vi "Online Spectrogram Monitoring (Simulated).vi"() -> ()   [LabVIEW 2023]
doc: "This example continuously simulates a signal and computes the real-time STFT spectrogram with the TFA Online STFT Spectrogram VI.\n\n<b>Instructions:</b>\n1) Run this VI.\n2) Observe the <b>Spectrogram</b>.\n3) Browse the Block Diagram of this example to learn how to configure the charts."
uses:
  <vilib>/addons/Time Frequency Analysis/Spectrogram.llb/TFA Online STFT Spectrogram (Real).vi
  <vilib>/addons/Time Frequency Analysis/_control.llb/TFA Configure Spectrogram Indicator (Predefined Color Table).vi
  <vilib>/addons/_Advanced Signal Processing/NI_AdvSigProcTFA.lvlib
panel:
  out "Signal":dbl[](graph)
  out "aspt-left-top":bool
  in  "Reset":bool
  in  "Stop":bool
  out "Spectrogram":dbl[][](graph)
  # "Overview: Continuously simulates a signal and computes the real-time STFT spectrogram with the TFA Online STFT Spectrogram VI.\nRequirements: LabVIEW Full Development System, Advanced Signal Processing Toolkit\nInstructions: \n1. Run this VI.\n2. Observe the Spectrogram.\n3. Browse the block diagram of this example to learn how to configure the charts.\n4. Click Stop to stop the VI."
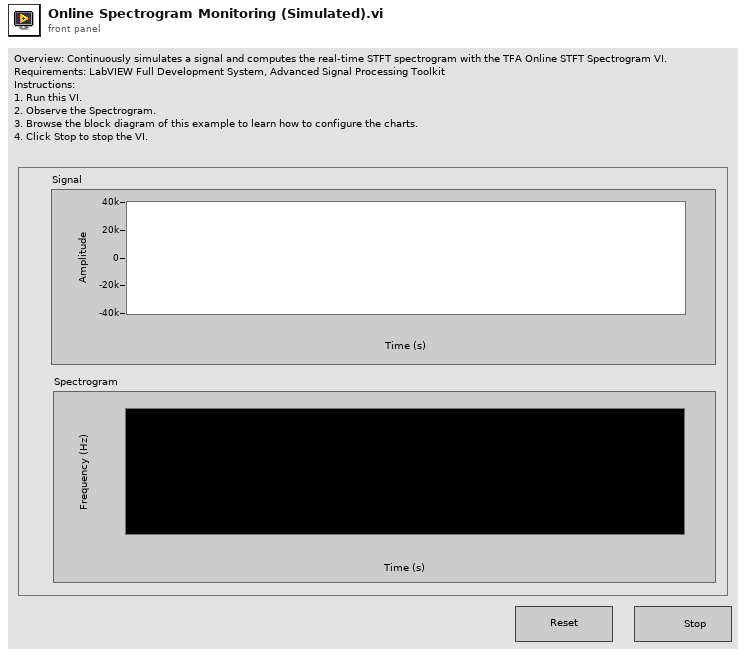
[diagram p1: front panel]
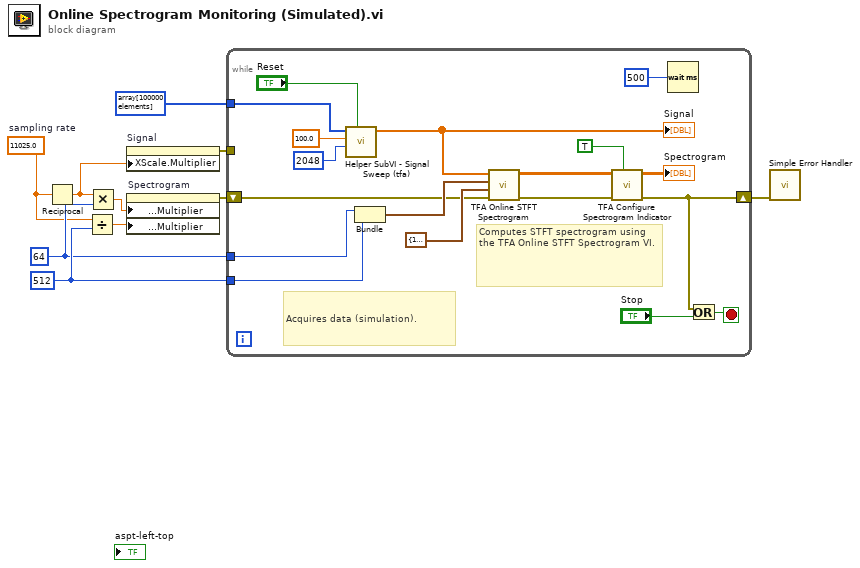
[diagram p0: block diagram]
diagram:
  w7 = 11025.0  # sampling rate
  w10 = 512 ("Frequency bins")
  w8 = 64 ("Time steps")
  n1 = Reciprocal(x=w7) -> (1/x=w4:dbl)
  n2 = Divide(x=w7, y=w10) -> (x/y=w9:dbl)
  n3 = Multiply(x=w4, y=w8) -> (x*y=w5:dbl)
  n4 = property on="Signal" class="WFChart (strict)"("XScale.Multiplier"=w4) -> (error out=w3:errorcluster)  [unwired: 2 in, 1 out]
  n5 = property on="Spectrogram" class="IntChart (strict)"("X Scale.Offset and Multiplier:Multiplier"=w5, "Y Scale.Offset and Multiplier:Multiplier"=w9) -> (error out=w6:errorcluster)  [unwired: 2 in, 1 out]
  n6 = while {
    tunnel: w8 -> [w24]
    tunnel: w10 -> [w23]
    tunnel: i16[] array[100000 elements] ("subarray") -> [w19]
    tunnel: w3 -> [_]
    shift-right: [w13] -> w2
    shift-left: w6 -> [w14]
    stop <- w11 stop-if-true
    # "Computes STFT spectrogram using the TFA Online STFT Spectrogram VI."
    # "Acquires data (simulation)."
    n7 = call "Helper SubVI - Signal Sweep (tfa).vi"("reset"="Reset", "length"=2048, "shift (%)"=100.0, "Signal in"=w19) -> ("Signal out"=w16:dbl[])  [unwired: 7 in]
    "Signal" <- w16
    n8 = Bundle("Time steps"=w24, "Frequency bins"=w23) -> (w27:cluster{"Time steps":i32, "Frequency bins":i32})  [unwired: 1 out]
    n9 = call-poly <vilib>:"TFA Online STFT Spectrogram.vi"("error in (no error)"=w14, "window info"=cluster{"type":i32, "length":i32} {"type"=1, "length"=512}, "time-frequency sampling info"=w27, "signal"=w16) -> ("error out"=w15:errorcluster, "spectrogram"=w26:dbl[][])  [unwired: 6 out]
    n10 = call-poly <vilib>:"TFA Configure Spectrogram Indicator.vi"("dB on? (F)"=TRUE ("dB? (F)"), "error in (no error)"=w15, "spectrogram"=w26) -> ("error out"=w13:errorcluster, "TF spectrogram indicator"=→"Spectrogram":dbl[][])  [unwired: 4 in, 3 out]
    n11 = Wait (ms)(milliseconds to wait=u32 500 ("millisecond multiple")) -> ()  [unwired: 1 out]
    n12 = Or(x=w13, y="Stop") -> (x .or. y?=w11:bool)
  }
  n13 = call <vilib>:"Simple Error Handler.vi"("error in (no error)"=w2) -> ()  [unwired: 4 in, 5 out]
